vi "A3-GPS-Decoder.vi"(2 "ASCII Hexidecimal String":string) -> (0 "Date (YYYYMMDD)":u32, 1 "Time (HHMMSS)":u32, 3 "Longitude (Deg)":dbl, 4 "Latitude (Deg)":dbl, 5 "AMSL (m)":u32, 6 "Velocity North (cm/s)":sgl, 7 "Velocity East (cm/s)":sgl, 8 "Velocity Down (cm/s)":sgl)   [LabVIEW 2018]
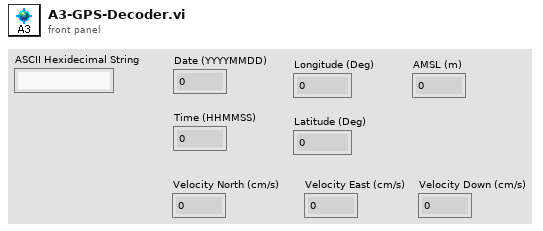
[diagram p1: front panel]
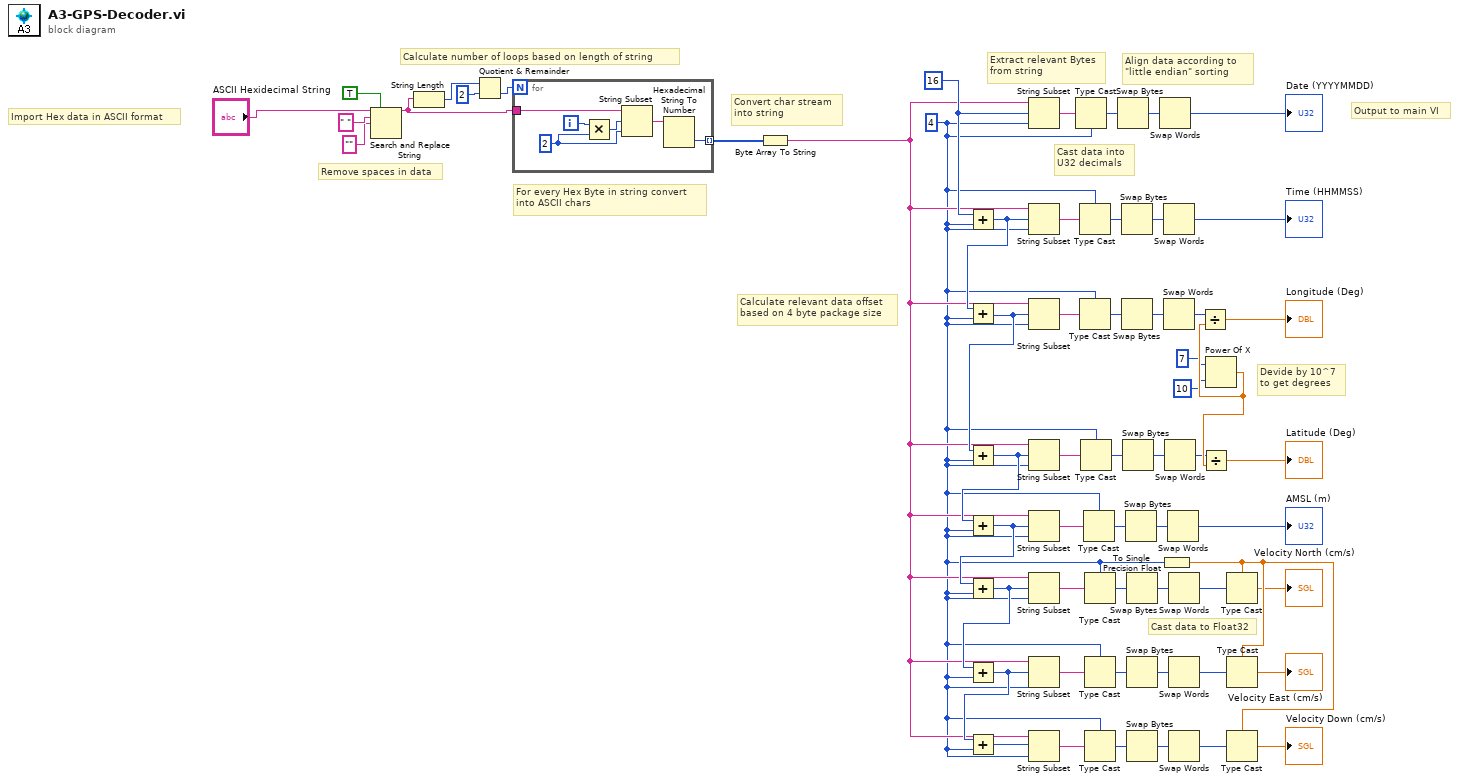
[diagram p0: block diagram]
diagram:
  w1 = u32 4 ("length (rest)")
  w21 = u32 16 ("offset (0)")
  # "Calculate relevant data offset \nbased on 4 byte package size"
  # "Cast data to Float32"
  # "Devide by 10^7 \nto get degrees"
  # "Output to main VI"
  # "Align data according to \n\"little endian\" sorting"
  # "Cast data into \nU32 decimals"
  # "Extract relevant Bytes \nfrom string"
  # "Convert char stream\ninto string"
  # "For every Hex Byte in string convert \ninto ASCII chars"
  # "Calculate number of loops based on length of string"
  # "Remove spaces in data"
  # "Import Hex data in ASCII format"
  n1 = Search and Replace String(replace all?=TRUE ("replace all? (F)"), input string="ASCII Hexidecimal String", search string=" ", replace string="" ("replace string (\"\")")) -> (result string=w4:string)  [unwired: 4 in, 3 out]
  n2 = String Length(string=w4) -> (length=w11:i32)
  n3 = Quotient & Remainder(x=w11, y=2) -> (floor(x/y)=w9:i32)  [unwired: 1 out]
  n4 = for {
    N: w9 -> [_]
    tunnel: w4 -> [w61]
    tunnel: [w62] -> w8 mode=indexing
    i -> [w65]
    w64 = 2 ("length (rest)")
    n5 = Multiply(x=w65, y=w64) -> (x*y=w66:i32)
    n6 = String Subset(string=w61, offset (0)=w66, length (rest)=w64) -> (substring=w63:string)
    n7 = Hexadecimal String To Number(string=w63) -> (number=w62:u32)  [unwired: 2 in, 1 out]
  }
  n8 = Byte Array To String(unsigned byte array=w8) -> (string=w3:string)
  n9 = Add(x=w21, y=w1) -> (x+y=w22:u32)
  n10 = Add(x=w22, y=w1) -> (x+y=w31:u32)
  n11 = Add(x=w31, y=w1) -> (x+y=w34:u32)
  n12 = Add(x=w34, y=w1) -> (x+y=w41:u32)
  n13 = Add(x=w41, y=w1) -> (x+y=w60:u32)
  n14 = Add(x=w60, y=w1) -> (x+y=w50:u32)
  n15 = Add(x=w50, y=w1) -> (x+y=w58:u32)
  n16 = String Subset(string=w3, offset (0)=w21, length (rest)=w1) -> (substring=w12:string)
  n17 = String Subset(string=w3, offset (0)=w22, length (rest)=w1) -> (substring=w51:string)
  n18 = String Subset(string=w3, offset (0)=w31, length (rest)=w1) -> (substring=w52:string)
  n19 = String Subset(string=w3, offset (0)=w34, length (rest)=w1) -> (substring=w53:string)
  n20 = String Subset(string=w3, offset (0)=w41, length (rest)=w1) -> (substring=w54:string)
  n21 = String Subset(string=w3, offset (0)=w60, length (rest)=w1) -> (substring=w55:string)
  n22 = String Subset(string=w3, offset (0)=w50, length (rest)=w1) -> (substring=w56:string)
  n23 = String Subset(string=w3, offset (0)=w58, length (rest)=w1) -> (substring=w57:string)
  n24 = Type Cast(type=w1, x=w12) -> (*(type *) &x=w14:u32)
  n25 = Type Cast(type=w1, x=w51) -> (*(type *) &x=w17:u32)
  n26 = Type Cast(type=w1, x=w52) -> (*(type *) &x=w20:u32)
  n27 = Type Cast(type=w1, x=w53) -> (*(type *) &x=w28:u32)
  n28 = Type Cast(type=w1, x=w54) -> (*(type *) &x=w35:u32)
  n29 = Type Cast(type=w1, x=w55) -> (*(type *) &x=w38:u32)
  n30 = Type Cast(type=w1, x=w56) -> (*(type *) &x=w43:u32)
  n31 = Type Cast(type=w1, x=w57) -> (*(type *) &x=w47:u32)
  n32 = Swap Bytes(anything=w14) -> (byte swapped=w13:u32)
  n33 = Swap Bytes(anything=w17) -> (byte swapped=w16:u32)
  n34 = Swap Bytes(anything=w20) -> (byte swapped=w19:u32)
  n35 = Swap Bytes(anything=w28) -> (byte swapped=w27:u32)
  n36 = Swap Bytes(anything=w35) -> (byte swapped=w33:u32)
  n37 = Swap Bytes(anything=w38) -> (byte swapped=w37:u32)
  n38 = Swap Bytes(anything=w43) -> (byte swapped=w42:u32)
  n39 = Swap Bytes(anything=w47) -> (byte swapped=w46:u32)
  n40 = Swap Words(1:w13) -> (0:→"Date (YYYYMMDD)":u32)
  n41 = To Single Precision Float(number=w1) -> (single precision float=w59:sgl)
  n42 = Swap Words(1:w16) -> (0:→"Time (HHMMSS)":u32)
  n43 = Swap Words(1:w19) -> (0:w25:u32)
  n44 = Swap Words(1:w27) -> (0:w29:u32)
  n45 = Swap Words(1:w33) -> (0:→"AMSL (m)":u32)
  n46 = Swap Words(1:w37) -> (0:w40:u32)
  n47 = Swap Words(1:w42) -> (0:w45:u32)
  n48 = Swap Words(1:w46) -> (0:w49:u32)
  n49 = Power Of X(1:10 ("x"), 2:7 ("y")) -> (0:w32:dbl)
  n50 = Divide(x=w25, y=w32) -> (x/y=→"Longitude (Deg)":dbl)
  n51 = Divide(x=w29, y=w32) -> (x/y=→"Latitude (Deg)":dbl)
  n52 = Type Cast(type=w59, x=w40) -> (*(type *) &x=→"Velocity North (cm/s)":sgl)
  n53 = Type Cast(type=w59, x=w45) -> (*(type *) &x=→"Velocity East (cm/s)":sgl)
  n54 = Type Cast(type=w59, x=w49) -> (*(type *) &x=→"Velocity Down (cm/s)":sgl)
